vi "PXI8431_com.vi"(10 "Slot":i32=6) -> ()   [LabVIEW 2017]
doc: "Use this template to build a producer/consumer design pattern with events to produce queue items. Use this design pattern instead of the User Interface Event Handler pattern for user interfaces when you want to execute code asynchronously in response to an event without slowing the user interface responsiveness."
uses:
  Hardware/Serial/Serial - Settings.ctl
  controls/FS_PXI8431com.ctl
panel:
  in  "Select Port":u16(ring)
  in  "Serial Settings":T1={"baud rate"=9600, "data bits"=8, "parity"=enum."None", "stop bits"=10, "flow control"=0} {"flow control" items=["None"=0, "XON/XOFF"=1, "RTS/CTS"=2, "DTR/DSR"=4]; "stop bits" items=["1.0"=10, "1.5"=15, "2.0"=20]; "data bits" min=5 max=8 step=1; "baud rate" items=["75"=75, "110"=110, "134"=134, "150"=150, "300"=300, "600"=600, "1200"=1200, "1800"=1800, "2400"=2400, "4800"=4800, "7200"=7200, "9600"=9600, "14400"=14400, "19200"=19200, "28800"=28800, "38400"=38400, "56000"=56000, "57600"=57600, "115200"=115200, "128000"=128000, "230400"=230400]}
  in  "OK":bool
  out "数据":string
  in  "命令":string
  # "PXI-8341串口通讯"
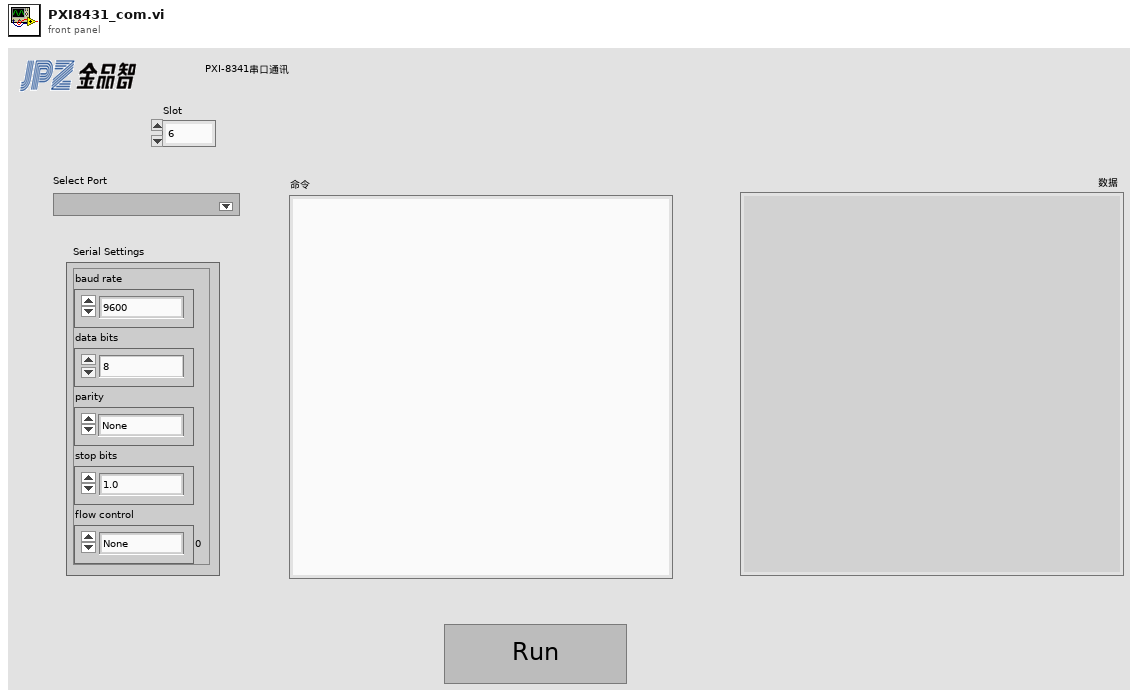
[diagram p1: front panel]
types:
  T1 = typedef "Serial - Settings.ctl" = cluster{"baud rate":u32, "data bits":u16, "parity":enum16{"None", "Odd", "Even", "Mark", "Space"}, "stop bits":u16, "flow control":u16}
  T2 = typedef "FS_PXI8431com.ctl" = enum16{"Initialize", "Select Slot", "Run Com", "Config", "Set Xon/Xoff", "Set TermChar", "Write Command", "Read Data", "Release Port"}
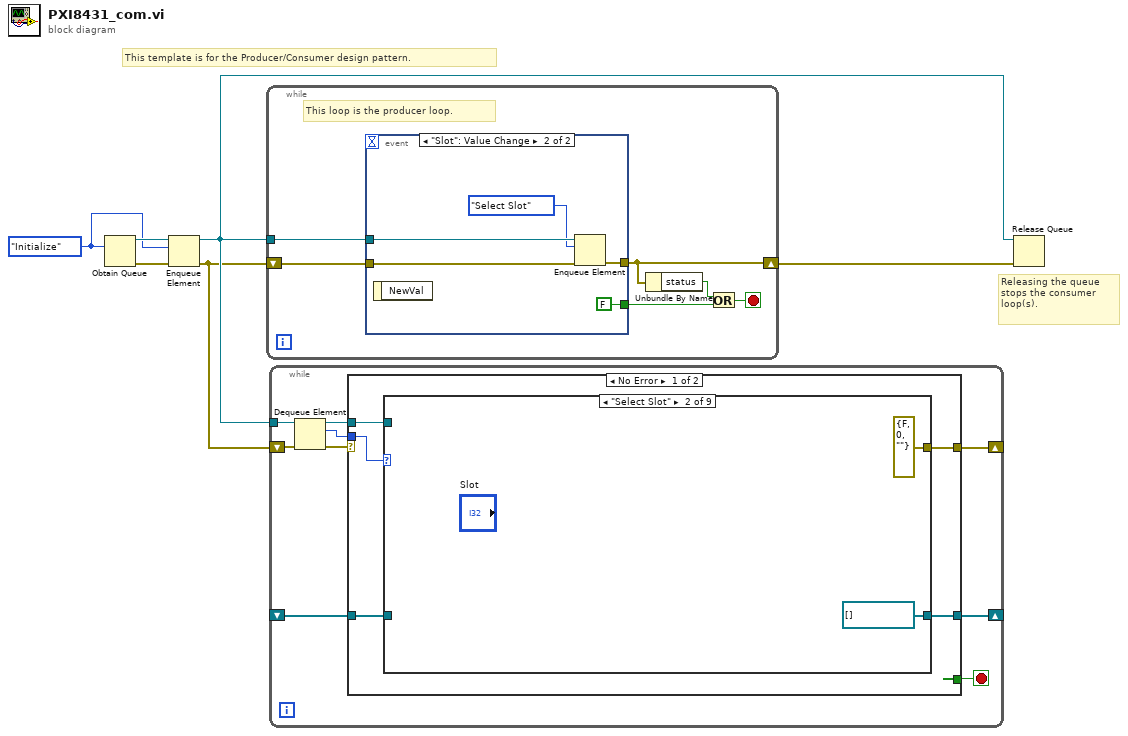
[diagram p0: block diagram]
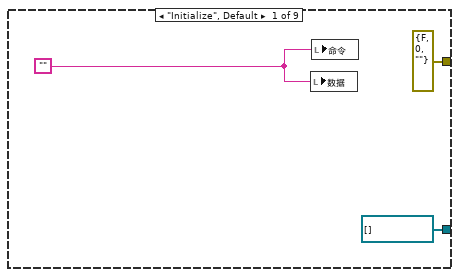
[diagram p2: hidden frame]
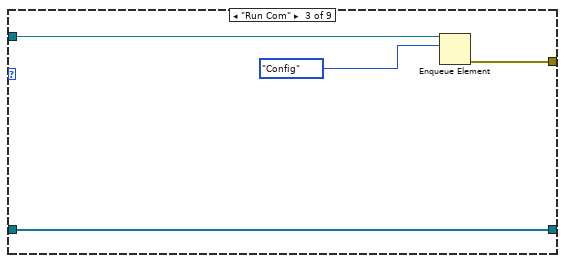
[diagram p3: hidden frame]
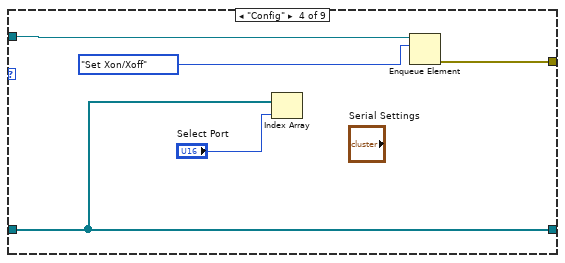
[diagram p4: hidden frame]
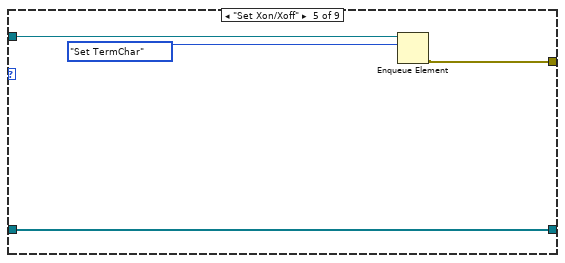
[diagram p5: hidden frame]
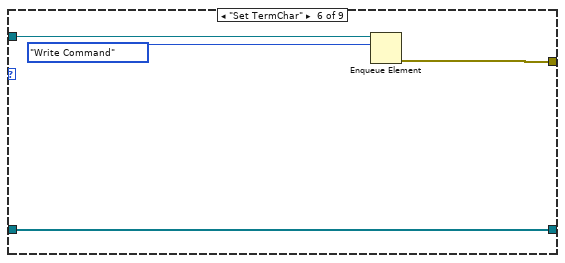
[diagram p6: hidden frame]
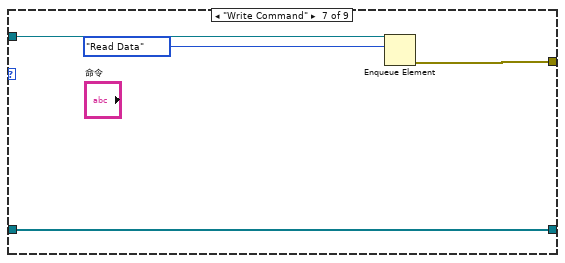
[diagram p7: hidden frame]
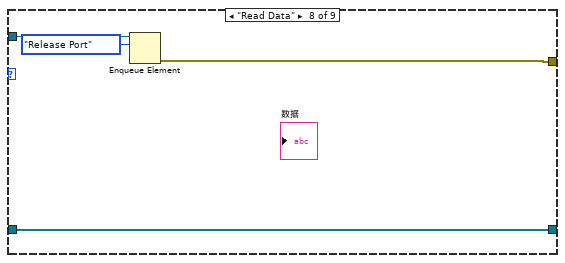
[diagram p8: hidden frame]
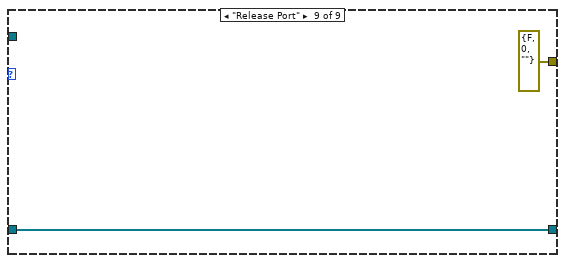
[diagram p9: hidden frame]
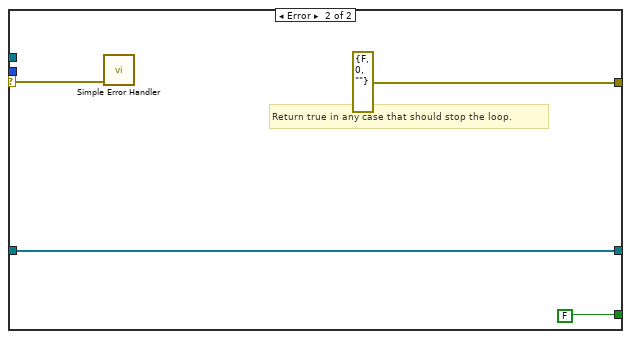
[diagram p10: hidden frame]
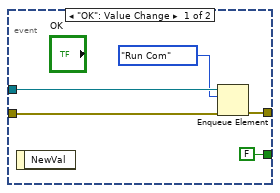
[diagram p11: hidden frame]
diagram:
  w2 = FS_PXI8431com."Initialize"
  # "Releasing the queue stops the consumer loop(s)."
  # "This template is for the Producer/Consumer design pattern."
  n1 = Obtain Queue(element data type=w2) -> (queue out=w5:refnum<queue>, error out=w3:errorcluster)  [unwired: 4 in, 1 out]
  n2 = Enqueue Element(queue=w5, element=w2, error in (no error)=w3) -> (queue out=w4:refnum<queue>, error out=w1:errorcluster)  [unwired: 1 in, 1 out]
  n3 = while {
    shift-right: [w8] -> w6
    shift-left: w1 -> [w11]
    tunnel: w4 -> [w12]
    stop <- w9 stop-if-true
    # "This loop is the producer loop."
    n4 = event shown="[1] \"Slot\": Value Change" {
      selector: _ -> [_ _]
      dyn-events: _ -> [_ _]
      timeout: _ -> [_ _]
      tunnel: w12 -> [w17 w22]
      tunnel: w11 -> [w16 w21]
      tunnel: [w15 w20] -> w8
      tunnel: [FALSE ("stop") FALSE ("stop")] -> w10
      event "OK": Value Change {
        n5 = event-data() -> ()  [unwired: 1 in, 1 out]
        n6 = Enqueue Element(queue=w17, element=FS_PXI8431com."Run Com", error in (no error)=w16) -> (error out=w15:errorcluster)  [unwired: 1 in, 2 out]
      }
      event "Slot": Value Change {
        n7 = event-data() -> ()  [unwired: 1 in, 1 out]
        n8 = Enqueue Element(queue=w22, element=FS_PXI8431com."Select Slot", error in (no error)=w21) -> (error out=w20:errorcluster)  [unwired: 1 in, 2 out]
      }
    }
    n9 = Unbundle By Name(w8) -> ("status"=w7:bool)
    n10 = Or(x=w7, y=w10) -> (x .or. y?=w9:bool)
  }
  n11 = while {
    tunnel: w4 -> [w31]
    shift-right: [w26] -> _
    shift-left: w1 -> [w25]
    shift-right: [w24] -> _
    shift-left: _ -> [w23]
    stop <- w28 stop-if-true
    n12 = Dequeue Element(queue=w31, error in (no error)=w25) -> (queue out=w27:refnum<queue>, element=w29:T2, error out=w30:errorcluster)  [unwired: 1 in, 1 out]
    n13 = case shown="No Error" w30 {
      selector: w30 -> [_ w70]
      tunnel: w29 -> [w36 _]
      tunnel: [_ FALSE] -> w28
      tunnel: w27 -> [w35 _]
      tunnel: [w34 errorcluster {"status"=FALSE, "code"=0, "source"=""} ("error out")] -> w26
      tunnel: [w33 w69] -> w24
      tunnel: w23 -> [w32 w69]
      frame No Error {
        n14 = case shown="\"Select Slot\"" w36 {
          tunnel: w35 -> [_ _ w45 w49 w54 w58 w62 w66 _]
          tunnel: [errorcluster {"status"=FALSE, "code"=0, "source"=""} ("error out") errorcluster {"status"=FALSE, "code"=0, "source"=""} ("error out") w44 w46 w51 w55 w59 w63 errorcluster {"status"=FALSE, "code"=0, "source"=""} ("error out")] -> w34
          tunnel: [refnum<visa-resource-name>[] [] ("VISA Ref") refnum<visa-resource-name>[] [] ("VISA Ref") w42 w47 w52 w56 w60 w64 w68] -> w33
          tunnel: w32 -> [_ _ w42 w47 w52 w56 w60 w64 w68]
          frame "Initialize", Default {
            w38 = ""
            n15 = local write "数据"(w38) -> ()
            n16 = local write "命令"(w38) -> ()
          }
          frame "Select Slot" {
          }
          frame "Run Com" {
            n17 = Enqueue Element(queue=w45, element=FS_PXI8431com."Config") -> (error out=w44:errorcluster)  [unwired: 2 in, 2 out]
          }
          frame "Config" {
            n18 = Index Array(array=w47, index="Select Port") -> ()  [unwired: 1 out]
            n19 = Enqueue Element(queue=w49, element=FS_PXI8431com."Set Xon/Xoff") -> (error out=w46:errorcluster)  [unwired: 2 in, 2 out]
          }
          frame "Set Xon/Xoff" {
            n20 = Enqueue Element(queue=w54, element=FS_PXI8431com."Set TermChar") -> (error out=w51:errorcluster)  [unwired: 2 in, 2 out]
          }
          frame "Set TermChar" {
            n21 = Enqueue Element(queue=w58, element=FS_PXI8431com."Write Command") -> (error out=w55:errorcluster)  [unwired: 2 in, 2 out]
          }
          frame "Write Command" {
            n22 = Enqueue Element(queue=w62, element=FS_PXI8431com."Read Data") -> (error out=w59:errorcluster)  [unwired: 2 in, 2 out]
          }
          frame "Read Data" {
            n23 = Enqueue Element(queue=w66, element=FS_PXI8431com."Release Port") -> (error out=w63:errorcluster)  [unwired: 2 in, 2 out]
          }
          frame "Release Port" {
          }
        }
      }
      frame Error {
        # "Return true in any case that should stop the loop."
        n24 = call <vilib>:"Simple Error Handler.vi"("error in (no error)"=w70) -> ()  [unwired: 4 in, 5 out]
      }
    }
  }
  n25 = Release Queue(queue=w4, error in (no error)=w6) -> ()  [unwired: 1 in, 3 out]
